vi "handshake_response.vi"(8 "error in (no error)":errorcluster, 11 "response":string) -> (0 "error out":errorcluster, 3 "value":variant)   [LabVIEW 2017, in "rethinkdb.lvlib"]
uses:
  rethinkdb.lvlib
  914ac796-27b2-451e-b7e8-bb850beead6e.vi
  69571172-70b3-47df-8e30-834d8fd0c3c5.vi
  d77eb173-89ea-478a-9aed-886234024754.vi
  json_get_names.vi
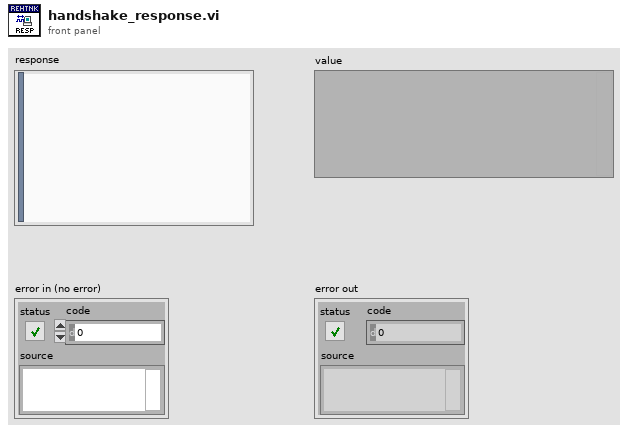
[diagram p1: front panel]
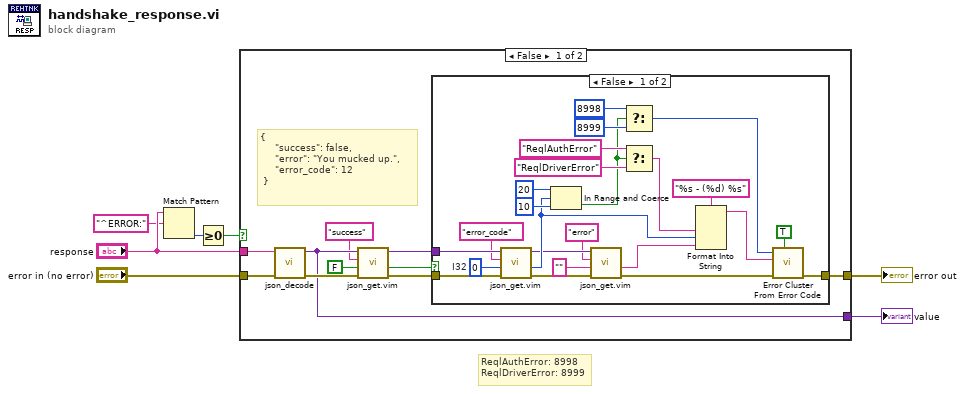
[diagram p0: block diagram]
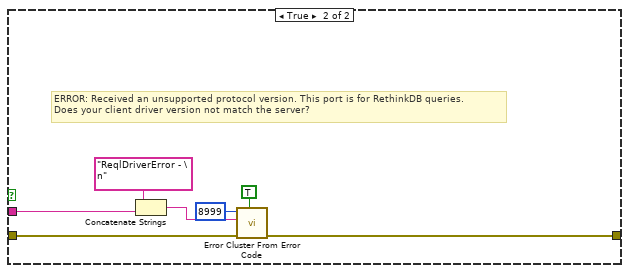
[diagram p3: hidden frame]
diagram:
  # "ReqlAuthError: 8998\nReqlDriverError: 8999"
  n1 = Match Pattern(string="response", regular expression="^ERROR:") -> (offset past match=w3:i32)  [unwired: 1 in, 3 out]
  n2 = Greater Or Equal To 0?(x=w3) -> (x >= 0?=w2:bool)
  n3 = case shown="False" w2 {
    tunnel: "error in (no error)" -> [w16 w46]
    tunnel: "response" -> [w15 w44]
    tunnel: [w17 w45] -> w4
    tunnel: [w13 _] -> w1
    frame False {
      # "{\n     \"success\": false,\n     \"error\": \"You mucked up.\",\n     \"error_code\": 12\n }"
      n4 = call "json_decode.vi"("error in (no error)"=w16, "json"=w15) -> ("error out"=w14:errorcluster, "variant"=w13:variant)  [unwired: 8 in]
      n5 = call "json_get.vim"("error in (no error)"=w14, "default"=FALSE, "name"="success" ("key"), "variant in"=w13) -> ("error out"=w10:errorcluster, "value"=w9:bool, "variant out"=w8:variant)  [unwired: 4 in, 1 out]
      n6 = case shown="False" w9 {
        tunnel: w10 -> [w28 w42]
        tunnel: w8 -> [w27 _]
        tunnel: [w38 w42] -> w17
        frame False {
          w26 = 0  # I32
          n7 = call "json_get.vim"("error in (no error)"=w28, "default"=w26, "name"="error_code" ("key"), "variant in"=w27) -> ("error out"=w23:errorcluster, "value"=w25:i32, "variant out"=w22:variant)  [unwired: 4 in, 1 out]
          n8 = In Range and Coerce(upper limit=20, x=w25, lower limit=10) -> (In Range?=w30:bool)  [unwired: 1 out]
          n9 = call "json_get.vim"("error in (no error)"=w23, "default"="", "name"="error" ("key"), "variant in"=w22) -> ("error out"=w19:errorcluster, "value"=w18:string)  [unwired: 4 in, 2 out]
          n10 = Select(t=8998 ("error code (0)"), s=w30, f=8999 ("error code (0)")) -> (s? t:f=w29:i32)
          n11 = Select(t="ReqlAuthError", s=w30, f="ReqlDriverError") -> (s? t:f=w33:string)
          n12 = Format Into String(format string="%s - (%d) %s" ("error message (\"\")"), w33, w25, w18) -> (resulting string=w34:string)  [unwired: 2 in, 1 out]
          n13 = call <vilib>:"Error Cluster From Error Code.vi"("show call chain? (False)"=TRUE, "error in (no error)"=w19, "error message (\"\")"=w34, "error code (0)"=w29) -> ("error out"=w38:errorcluster)  [unwired: 5 in]
        }
        frame True {
        }
      }
    }
    frame True {
      # "ERROR: Received an unsupported protocol version. This port is for RethinkDB queries. \nDoes your client driver version not match the server?"
      n14 = Concatenate Strings("ReqlDriverError - \n" ("error message (\"\")"), w44) -> (w43:string)
      n15 = call <vilib>:"Error Cluster From Error Code.vi"("show call chain? (False)"=TRUE, "error in (no error)"=w46, "error message (\"\")"=w43, "error code (0)"=8999) -> ("error out"=w45:errorcluster)  [unwired: 5 in]
    }
  }
  "error out" <- w4
  "value" <- w1
